vi "three_button.vi"(7 "callee":refnum<vi>, 8 "error in (no error)":errorcluster, 10 "configuration":T2, 11 "v1 in":refnum<class "v1.lvclass">) -> (0 "error out":errorcluster, 2 "dialog_selection":T1, 3 "v1 out":refnum<class "v1.lvclass">)   [LabVIEW 2015, in "lv-dialog.lvlib" / "v1.lvlib" / "v1.lvclass"]
uses:
  v1.lvclass
  _controls/selection.ctl
  v1.lvlib
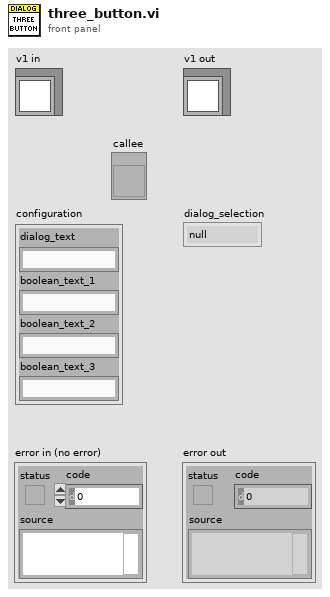
[diagram p1: front panel]
types:
  T1 = typedef "lv-dialog.lvlib/v1.lvlib/selection.ctl" = enum16{"null", "panel_closed", "button_1", "button_2", "button_3", "cancelled"}
  T2 = cluster{"dialog_text":string, "boolean_text_1":string, "boolean_text_2":string, "boolean_text_3":string}
  T3 = enum16{"Left Button", "Center Button", "Right Button", "Window Close"}
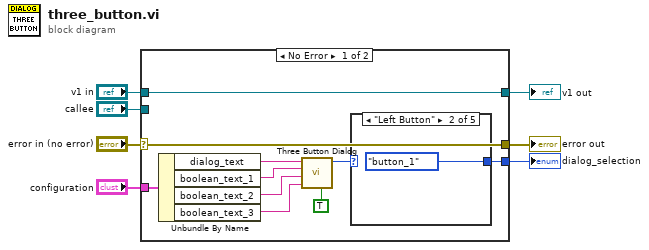
[diagram p0: block diagram]
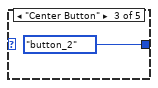
[diagram p3: hidden frame]
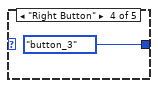
[diagram p4: hidden frame]
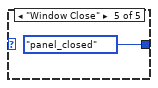
[diagram p5: hidden frame]
diagram:
  n1 = case shown="No Error" "error in (no error)" {
    selector: "error in (no error)" -> [w15 w23]
    tunnel: [w15 w23] -> w6
    tunnel: [w17 w22] -> w4
    tunnel: "v1 in" -> [w17 w22]
    tunnel: "configuration" -> [w16 _]
    tunnel: "callee" -> [_ _]
    tunnel: [w8 _] -> w1
    frame No Error {
      n2 = Unbundle By Name(w16) -> ("dialog_text"=w14:string, "boolean_text_1"=w13:string, "boolean_text_2"=w12:string, "boolean_text_3"=w11:string)
      n3 = call <vilib>:"Three Button Dialog.vi"("Allow user to close window? (TRUE)"=TRUE, "Right Button Text (\"Cancel\")"=w11, "Center Button Text (\"No\")"=w12, "Left Button Text (\"Yes\")"=w13, "message"=w14) -> ("Which Button?"=w9:T3)  [unwired: 6 in]
      n4 = case shown="\"Left Button\"" w9 {
        tunnel: [_ selection."button_1" ("dialog_selection") selection."button_2" ("dialog_selection") selection."button_3" ("dialog_selection") selection."panel_closed" ("dialog_selection")] -> w8
        frame Default {
        }
        frame "Left Button" {
        }
        frame "Center Button" {
        }
        frame "Right Button" {
        }
        frame "Window Close" {
        }
      }
    }
    frame Error {
    }
  }
  "error out" <- w6
  "v1 out" <- w4
  "dialog_selection" <- w1
